vi "Get Cargo Capacity.vi"(8 "error in":errorcluster, 11 "vehicle":refnum<class "Vehicle.lvclass">) -> (0 "error out":errorcluster, 2 "cargo capacity":dbl)   [LabVIEW 2013, in "Vehicle.lvclass"]
doc: "This VI is an example of a dynamic member VI. It returns the cargo capacity for the vehicle."
uses:
  Vehicle.lvclass
  Vehicle.lvclass/Vehicle.ctl
panel:
  # "This VI is an example of a dynamic member VI."
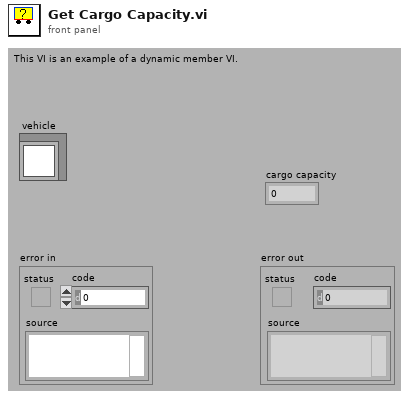
[diagram p1: front panel]
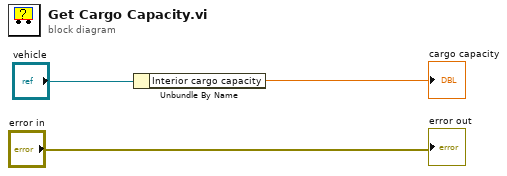
[diagram p0: block diagram]
diagram:
  n1 = Unbundle By Name("vehicle") -> ("Interior cargo capacity"=→"cargo capacity":dbl)
  "error out" <- "error in"
